vi "Timing Sort by Priority.vi"() -> ()   [LabVIEW 2017]
uses:
  Source/Engine/Classes/Transfer/DSF.Engine.Transfer.lvclass
  Source/DSF Configuration API/1.0.0/Public/Controls/DSF Direction.ctl
  Source/Engine/Classes/Timing/DSF.Engine.Timing.lvclass/DSF.Engine.Timing.ctl
  Source/Engine/Classes/Transfer/DSF.Engine.Transfer Group.lvclass/DSF.Engine.Transfer Group.ctl
  Source/Engine/Classes/Timing/DSF.Engine.Timing.lvclass
  Source/Engine/Classes/Transfer/DSF.Engine.Transfer Group.lvclass
  Source/DSF Configuration API/1.0.0/DSF Configuration API.lvlib
panel:
  out "group post-sort":u64[](array[numeric])
  out "post-sort":u64[](array[numeric])
  out "pre-sort":u64[](array[numeric])
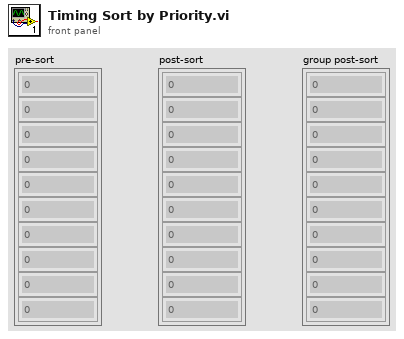
[diagram p1: front panel]
types:
  T1 = typedef "DSF Configuration API.lvlib/DSF Direction.ctl" = enum8{"Tx", "Rx"}
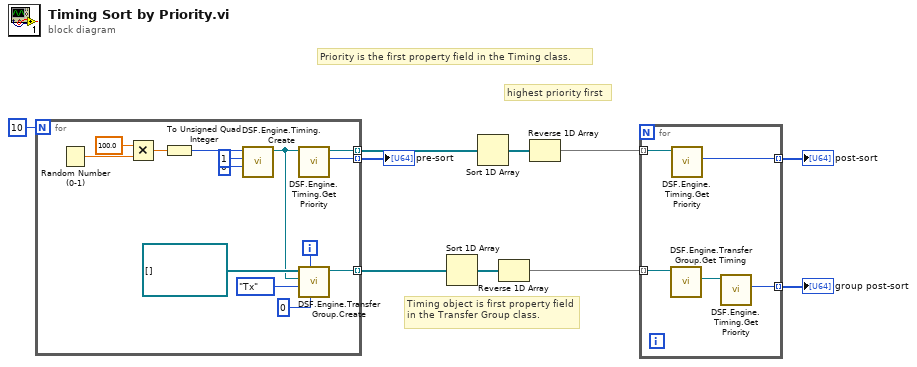
[diagram p0: block diagram]
diagram:
  # "Timing object is first property field in the Transfer Group class."
  # "highest priority first"
  # "Priority is the first property field in the Timing class."
  n1 = for {
    N: 10 -> [_]
    tunnel: [w18] -> w9 mode=indexing
    tunnel: [w17] -> w8 mode=indexing
    tunnel: [w12] -> w3 mode=indexing
    i -> [w16]
    n2 = Random Number (0-1)() -> (number: 0 to 1=w24:dbl)
    n3 = Multiply(x=100.0, y=w24) -> (x*y=w22:dbl)
    n4 = To Unsigned Quad Integer(1:w22) -> (0:w21:u64)
    n5 = call "DSF.Engine.Timing.Create.vi"("Offset"=u64 0, "Decimation"=u64 1, "Priority"=w21) -> ("Timing"=w13:refnum<class "DSF.Engine.Timing.lvclass">)  [unwired: 7 in, 1 out]
    n6 = call "DSF.Engine.Timing.Get Priority.vi"("Timing in"=w13) -> ("Priority"=w17:u64, "Timing out"=w18:refnum<class "DSF.Engine.Timing.lvclass">)  [unwired: 9 in]
    n7 = call "DSF.Engine.Transfer Group.Create.vi"("transceiver id"=0, "framework id"=w16, "Direction"=DSF_Direction."Tx", "Timing"=w13, "Transfers"=refnum<class "DSF.Engine.Transfer.lvclass">[] []) -> ("Transfer Group out"=w12:refnum<class "DSF.Engine.Transfer Group.lvclass">)  [unwired: 5 in, 1 out]
  }
  "pre-sort" <- w8
  n8 = Sort 1D Array(array=w3) -> (sorted array=w4:refnum<class "DSF.Engine.Transfer Group.lvclass">[])
  n9 = Sort 1D Array(array=w9) -> (sorted array=w6:refnum<class "DSF.Engine.Timing.lvclass">[])
  n10 = Reverse 1D Array(array=w4) -> (reversed array=w2:refnum<class "DSF.Engine.Transfer Group.lvclass">[])
  n11 = Reverse 1D Array(array=w6) -> (reversed array=w5:refnum<class "DSF.Engine.Timing.lvclass">[])
  n12 = for {
    tunnel: w5 -> [w29] mode=indexing
    tunnel: [w28] -> w7 mode=indexing
    tunnel: w2 -> [w27] mode=indexing
    tunnel: [w25] -> w1 mode=indexing
    n13 = call "DSF.Engine.Transfer Group.Get Timing.vi"("Transfer Group in"=w27) -> ("Timing"=w26:refnum<class "DSF.Engine.Timing.lvclass">)  [unwired: 9 in, 1 out]
    n14 = call "DSF.Engine.Timing.Get Priority.vi"("Timing in"=w29) -> ("Priority"=w28:u64)  [unwired: 9 in, 1 out]
    n15 = call "DSF.Engine.Timing.Get Priority.vi"("Timing in"=w26) -> ("Priority"=w25:u64)  [unwired: 9 in, 1 out]
  }
  "post-sort" <- w7
  "group post-sort" <- w1
